vi "FW102C_control.vi"(3 "error in (no error)":errorcluster, 4 "Current Wavelength":dbl, 5 "FW102C in":i32) -> (0 "error out":errorcluster, 1 "Position":i32, 2 "FW102C out":i32)   [LabVIEW 2018]
uses:
  Other Libraries/Thorlabs_FW102C/Thorlabs_FW102C.lvlib
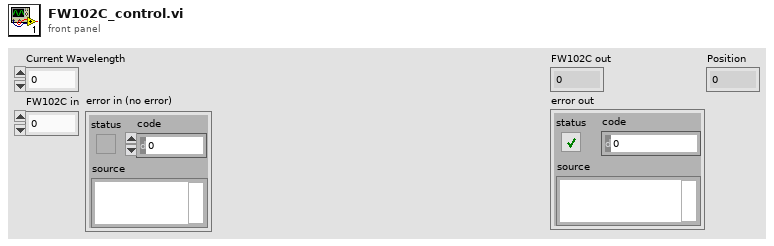
[diagram p1: front panel]
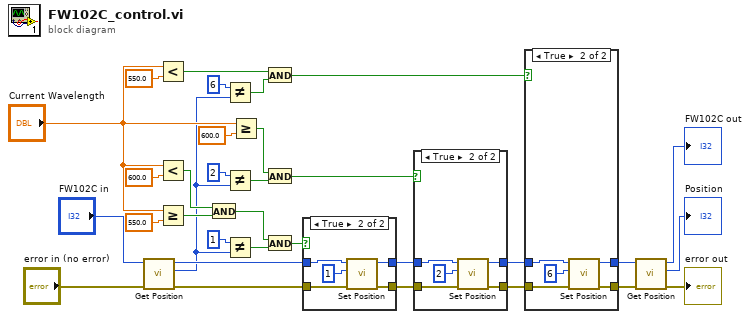
[diagram p0: block diagram]
diagram:
  n1 = call "Get Position.vi"("error in (no error)"="error in (no error)", "FW102C in"="FW102C in") -> ("error out"=w24:errorcluster, "Position"=w12:i32, "FW102C out"=w25:i32)  [unwired: 7 in]
  n2 = Less?(x="Current Wavelength", y=550.0) -> (x < y?=w10:bool)
  n3 = Less?(x="Current Wavelength", y=600.0) -> (x < y?=w31:bool)
  n4 = Greater Or Equal?(x="Current Wavelength", y=550.0) -> (x >= y?=w30:bool)
  n5 = And(x=w31, y=w30) -> (x .and. y?=w27:bool)
  n6 = Not Equal?(x=6, y=w12) -> (x != y?=w9:bool)
  n7 = Not Equal?(x=2, y=w12) -> (x != y?=w20:bool)
  n8 = Not Equal?(x=1, y=w12) -> (x != y?=w28:bool)
  n9 = Greater Or Equal?(x="Current Wavelength", y=600.0) -> (x >= y?=w21:bool)
  n10 = And(x=w10, y=w9) -> (x .and. y?=w8:bool)
  n11 = And(x=w21, y=w20) -> (x .and. y?=w17:bool)
  n12 = And(x=w27, y=w28) -> (x .and. y?=w26:bool)
  n13 = case shown="True" w26 {
    tunnel: w25 -> [w35 w40]
    tunnel: [w35 w39] -> w19
    tunnel: w24 -> [w34 w38]
    tunnel: [w34 w37] -> w18
    frame False {
    }
    frame True {
      n14 = call "Set Position.vi"("error in (no error)"=w38, "Position"=1, "FW102C in"=w40) -> ("error out"=w37:errorcluster, "FW102C out"=w39:i32)  [unwired: 7 in]
    }
  }
  n15 = case shown="True" w17 {
    tunnel: w19 -> [w42 w47]
    tunnel: [w42 w46] -> w16
    tunnel: w18 -> [w41 w45]
    tunnel: [w41 w44] -> w15
    frame False {
    }
    frame True {
      n16 = call "Set Position.vi"("error in (no error)"=w45, "Position"=2, "FW102C in"=w47) -> ("error out"=w44:errorcluster, "FW102C out"=w46:i32)  [unwired: 7 in]
    }
  }
  n17 = case shown="True" w8 {
    tunnel: w16 -> [w49 w54]
    tunnel: [w49 w53] -> w5
    tunnel: w15 -> [w48 w52]
    tunnel: [w48 w51] -> w3
    frame False {
    }
    frame True {
      n18 = call "Set Position.vi"("error in (no error)"=w52, "Position"=6, "FW102C in"=w54) -> ("error out"=w51:errorcluster, "FW102C out"=w53:i32)  [unwired: 7 in]
    }
  }
  n19 = call "Get Position.vi"("error in (no error)"=w3, "FW102C in"=w5) -> ("error out"=→"error out":errorcluster, "Position"=→"Position":i32, "FW102C out"=→"FW102C out":i32)  [unwired: 7 in]
